vi "HP 3326A (DUAL) Function Gen - SIMPLE.vi"(3 "Execute?":bool=TRUE, 4 "init cmd":string, 5 "Channel (0:A, 1:B)":i32, 7 "signal type (off:0)":u16(ring) items=["off", "sine", "square", "dc"], 8 "Phase (deg)":ext=1000000.0 format="%.3f", 9 "frequency (Hz)":ext=1000.0 format="%.3f", 10 "offset (V)":ext format="%.2f", 11 "amplitude (V)":ext=1.0 format="%.4f") -> (0 "cmd":string)   [LabVIEW 2014]
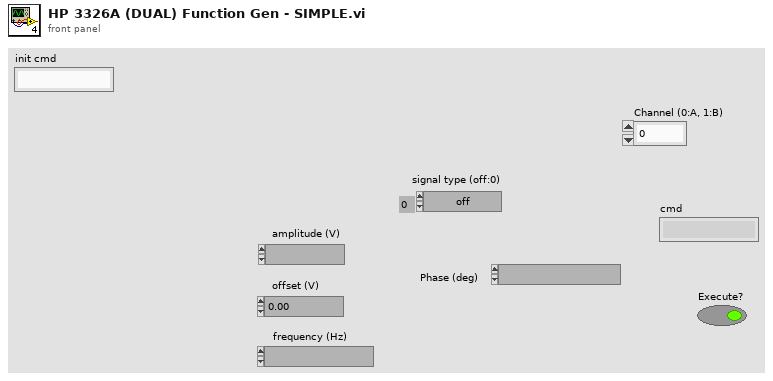
[diagram p1: front panel]
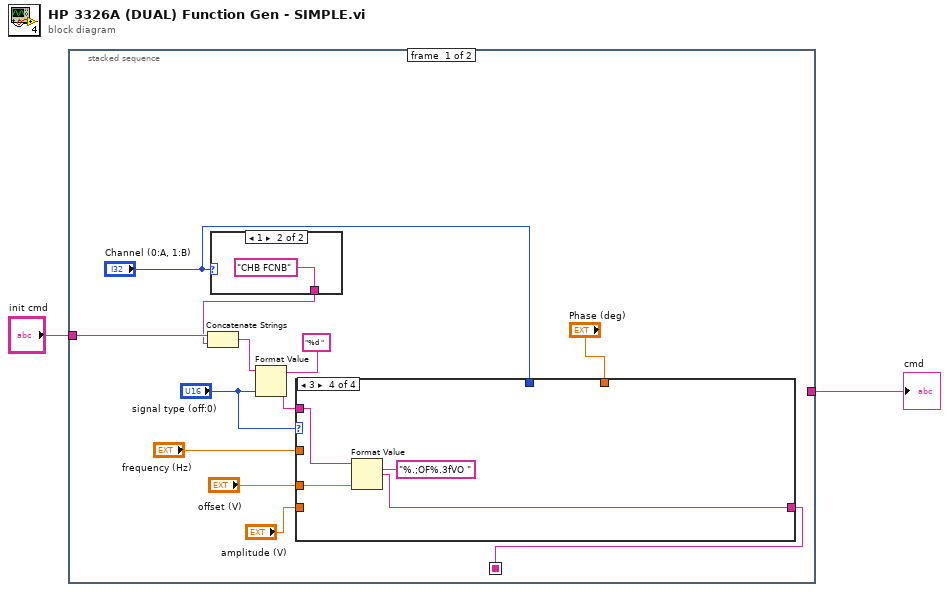
[diagram p0: block diagram]
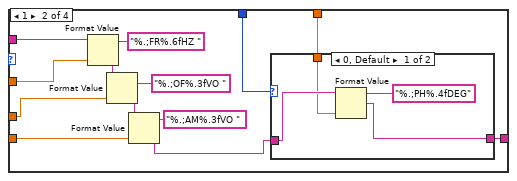
[diagram p3: hidden frame]
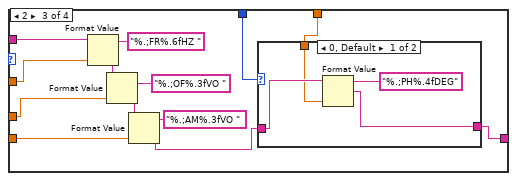
[diagram p5: hidden frame]
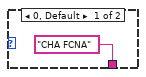
[diagram p7: hidden frame]
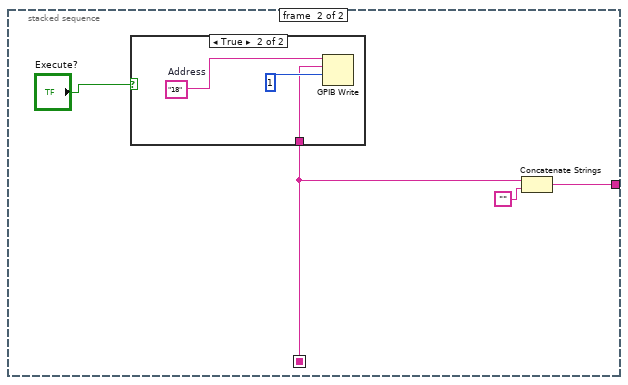
[diagram p8: hidden frame]
diagram:
  n1 = stacked-sequence {
    seq-local: [w3 _] -> [_ w58]
    tunnel: [_ w59] -> w2
    tunnel: "init cmd" -> [w12 _]
    frame #0 {
      n2 = case shown="1" "Channel (0:A, 1:B)" {
        tunnel: ["CHA FCNA" "CHB FCNB"] -> w11
        frame 0, Default {
        }
        frame 1 {
        }
      }
      n3 = Concatenate Strings(w12, w11) -> (w10:string)
      n4 = Format Value(string ("")=w10, format string="%d ", value (0)="signal type (off:0)") -> (output string=w13:string)
      n5 = case shown="3" "signal type (off:0)" {
        tunnel: w13 -> [w15 w23 w41 w54]
        tunnel: [w15 w17 w34 w52] -> w3
        tunnel: "offset (V)" -> [_ w22 w40 w53]
        tunnel: "amplitude (V)" -> [_ w21 w38 _]
        tunnel: "frequency (Hz)" -> [_ w20 w39 _]
        tunnel: "Channel (0:A, 1:B)" -> [_ w19 w35 _]
        tunnel: "Phase (deg)" -> [_ w16 w37 _]
        frame 0, Default {
        }
        frame 1 {
          n6 = Format Value(string ("")=w23, format string="%.;FR%.6fHZ ", value (0)=w20) -> (output string=w25:string)
          n7 = Format Value(string ("")=w25, format string="%.;OF%.3fVO ", value (0)=w22) -> (output string=w26:string)
          n8 = Format Value(string ("")=w26, format string="%.;AM%.3fVO ", value (0)=w21) -> (output string=w18:string)
          n9 = case shown="0, Default" w19 {
            tunnel: w18 -> [w31 w33]
            tunnel: [w30 w33] -> w17
            tunnel: w16 -> [w29 _]
            frame 0, Default {
              n10 = Format Value(string ("")=w31, format string="%.;PH%.4fDEG", value (0)=w29) -> (output string=w30:string)
            }
            frame 1 {
            }
          }
        }
        frame 2 {
          n11 = Format Value(string ("")=w41, format string="%.;FR%.6fHZ ", value (0)=w39) -> (output string=w43:string)
          n12 = Format Value(string ("")=w43, format string="%.;OF%.3fVO ", value (0)=w40) -> (output string=w44:string)
          n13 = Format Value(string ("")=w44, format string="%.;AM%.3fVO ", value (0)=w38) -> (output string=w36:string)
          n14 = case shown="0, Default" w35 {
            tunnel: w36 -> [w49 w51]
            tunnel: [w48 w51] -> w34
            tunnel: w37 -> [w47 _]
            frame 0, Default {
              n15 = Format Value(string ("")=w49, format string="%.;PH%.4fDEG", value (0)=w47) -> (output string=w48:string)
            }
            frame 1 {
            }
          }
        }
        frame 3 {
          n16 = Format Value(string ("")=w54, format string="%.;OF%.3fVO ", value (0)=w53) -> (output string=w52:string)
        }
      }
    }
    frame #1 {
      n17 = case shown="True" "Execute?" {
        tunnel: w58 -> [_ w62]
        frame False {
        }
        frame True {
          w63 = "18"  # Address
          n18 = GPIB Write(0:w63, 1:w62, 2:1) -> ()  [unwired: 1 in, 3 out]
        }
      }
      n19 = Concatenate Strings(w58, "") -> (w59:string)
    }
  }
  "cmd" <- w2
